vi "DLS_ERD Read.vi"(0 "GEA2 Reference In":refnum<k24>, 1 "Input Bit":T1, 2 "Co-efficient Data":T2, 5 "Standalone?":bool, 7 "GEA Inputs":T4 {"Destination" format="%.0x"; "Source" format="%.0x"}, 11 "Error In":errorcluster) -> (4 "GEA2 Reference Out":refnum<k24>, 6 "DLS ERD Data":T3, 8 "Result Q5 Tranformation":dbl, 15 "Error Out":errorcluster)   [LabVIEW 2016, in "TLMB.lvlib"]
doc: "This vi can be used to read ERD every 1 sec for user selected repeat counts."
uses:
  Projects/TLMB.lvlib
  Q:/Common/DLLs/GEA3/GeaCommunication.dll
  Common/DLLs/GEA3/GeaCommunication.dll
  Common/LabVIEW GEA2 Toolkit/LabVIEW_GEA2_Toolkit.lvlibp/type defs/Source_Destination.ctl
  Control/DLS ERD Data.ctl
  Common/LabVIEW GEA2 Toolkit/LabVIEW_GEA2_Toolkit.lvlibp/type defs/ERD Read Data In.ctl
  Common/LabVIEW GEA2 Toolkit/LabVIEW_GEA2_Toolkit.lvlibp/type defs/Data Type.ctl
  Common/LabVIEW GEA2 Toolkit/LabVIEW_GEA2_Toolkit.lvlibp
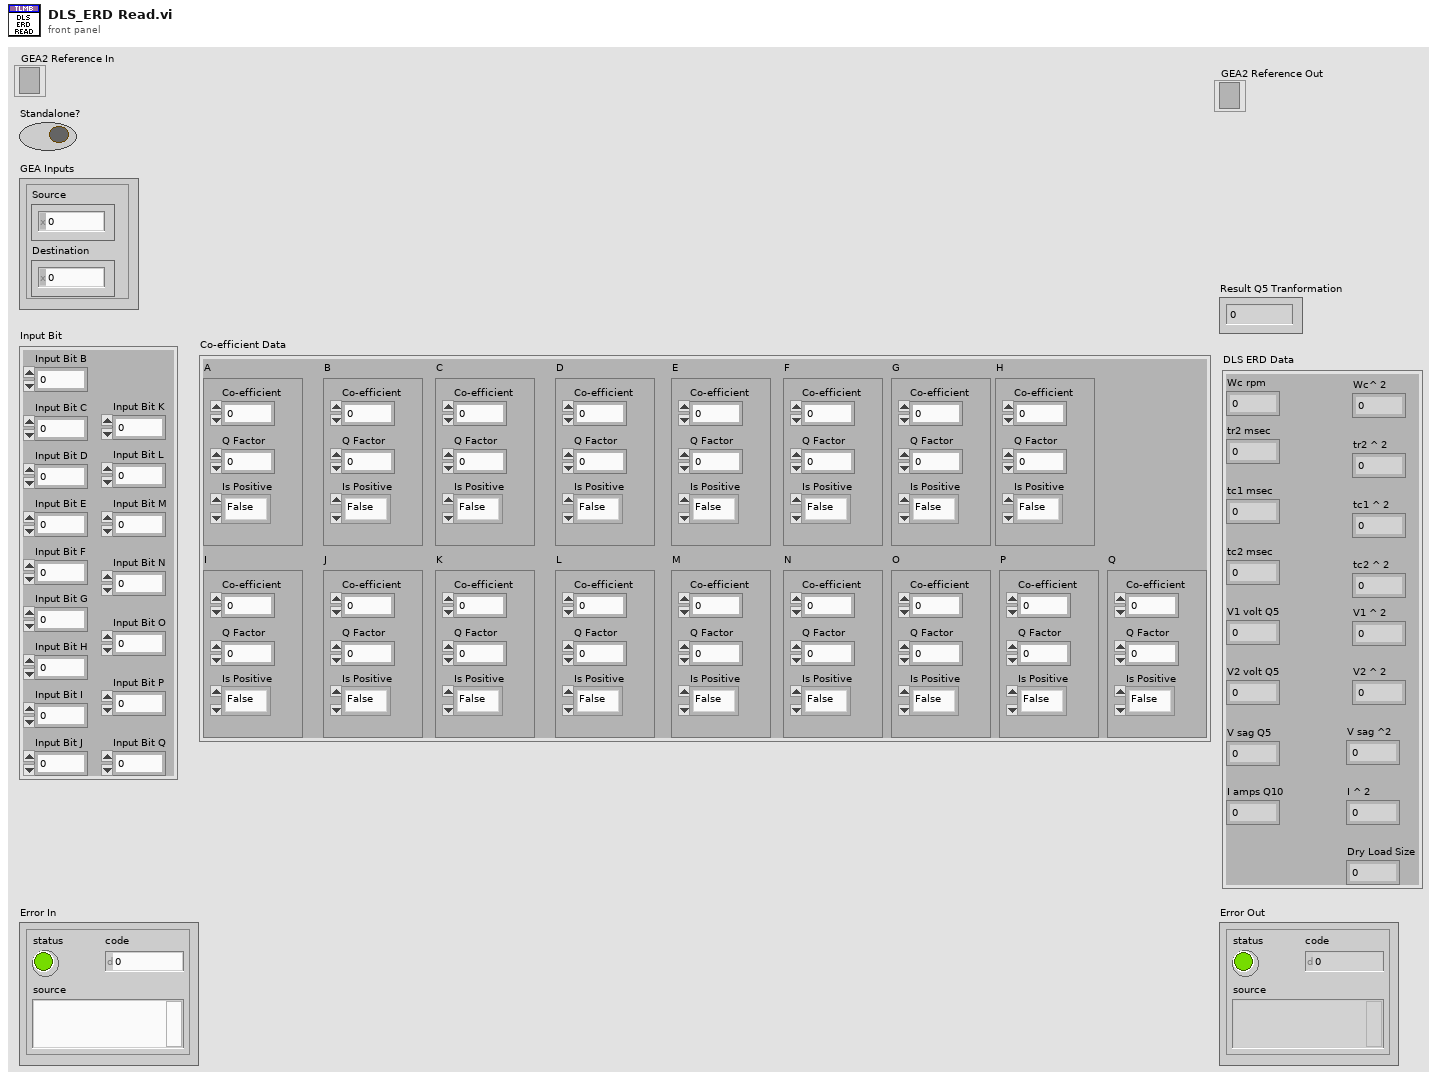
[diagram p1: front panel]
types:
  T1 = cluster{"Input Bit B":dbl, "Input Bit C":dbl, "Input Bit D":dbl, "Input Bit E":dbl, "Input Bit F":dbl, "Input Bit G":dbl, "Input Bit H":dbl, "Input Bit I":dbl, "Input Bit J":dbl, "Input Bit K":dbl, "Input Bit L":dbl, "Input Bit M":dbl, "Input Bit N":dbl, "Input Bit O":dbl, "Input Bit P":dbl, "Input Bit Q":dbl}
  T2 = cluster{"A":cluster{"Co-efficient":dbl, "Q Factor":dbl, "Is Positive":enum16{"False", "True"}}, "B":cluster{"Co-efficient":dbl, "Q Factor":dbl, "Is Positive":enum16{"False", "True"}}, "C":cluster{"Co-efficient":dbl, "Q Factor":dbl, "Is Positive":enum16{"False", "True"}}, "D":cluster{"Co-efficient":dbl, "Q Factor":dbl, "Is Positive":enum16{"False", "True"}}, "E":cluster{"Co-efficient":dbl, "Q Factor":dbl, "Is Positive":enum16{"False", "True"}}, "F":cluster{"Co-efficient":dbl, "Q Factor":dbl, "Is Positive":enum16{"False", "True"}}, "G":cluster{"Co-efficient":dbl, "Q Factor":dbl, "Is Positive":enum16{"False", "True"}}, "H":cluster{"Co-efficient":dbl, "Q Factor":dbl, "Is Positive":enum16{"False", "True"}}, "I":cluster{"Co-efficient":dbl, "Q Factor":dbl, "Is Positive":enum16{"False", "True"}}, "J":cluster{"Co-efficient":dbl, "Q Factor":dbl, "Is Positive":enum16{"False", "True"}}, "K":cluster{"Co-efficient":dbl, "Q Factor":dbl, "Is Positive":enum16{"False", "True"}}, "L":cluster{"Co-efficient":dbl, "Q Factor":dbl, "Is Positive":enum16{"False", "True"}}, "M":cluster{"Co-efficient":dbl, "Q Factor":dbl, "Is Positive":enum16{"False", "True"}}, "N":cluster{"Co-efficient":dbl, "Q Factor":dbl, "Is Positive":enum16{"False", "True"}}, "O":cluster{"Co-efficient":dbl, "Q Factor":dbl, "Is Positive":enum16{"False", "True"}}, "P":cluster{"Co-efficient":dbl, "Q Factor":dbl, "Is Positive":enum16{"False", "True"}}, "Q":cluster{"Co-efficient":dbl, "Q Factor":dbl, "Is Positive":enum16{"False", "True"}}}
  T3 = typedef "TLMB.lvlib/DLS ERD Data.ctl" = cluster{"Wc rpm":dbl, "tr2 msec":dbl, "tc1 msec":dbl, "tc2 msec":dbl, "V1 volt Q5":dbl, "V2 volt Q5":dbl, "I amps Q10":dbl, "Wc^ 2":dbl, "tr2 ^ 2":dbl, "tc1 ^ 2":dbl, "tc2 ^ 2":dbl, "V1 ^ 2":dbl, "V2 ^ 2":dbl, "I ^ 2":dbl, "V sag Q5":dbl, "V sag ^2":dbl, "Dry Load Size":dbl}
  T4 = typedef "LabVIEW_GEA2_Toolkit.lvlibp/Source_Destination.ctl" = cluster{"Source":u8, "Destination":u8}
  T5 = typedef "LabVIEW_GEA2_Toolkit.lvlibp/ERD Read Data In.ctl" = cluster{"ERD Number":u16, "Data Type":T6}
  T6 = typedef "LabVIEW_GEA2_Toolkit.lvlibp/Data Type.ctl" = enum16{"string", "boolean", "uint8_t", "uint16_t", "uint32_t", "uint64_t", "int8_t", "int16_t", "int32_t", "int64_t"}
  T7 = typedef "LabVIEW_GEA2_Toolkit.lvlibp/ERD Read Data Out.ctl" = cluster{"ERD Number":u16, "Data":string}
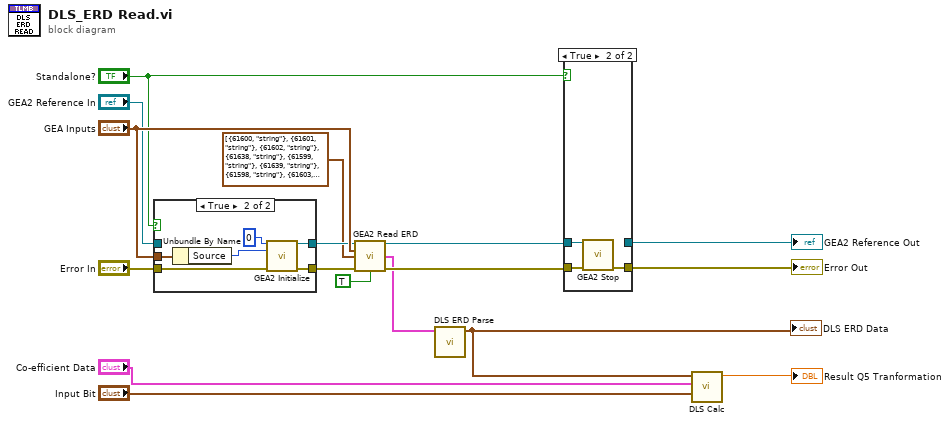
[diagram p0: block diagram]
diagram:
  n1 = case shown="True" "Standalone?" {
    tunnel: "Error In" -> [w18 w25]
    tunnel: [w18 w24] -> w12
    tunnel: "GEA2 Reference In" -> [w19 _]
    tunnel: [w19 w23] -> w11
    tunnel: "GEA Inputs" -> [_ w21]
    frame False {
    }
    frame True {
      n2 = Unbundle By Name(w21) -> ("Source"=w22:u8)
      n3 = call "GEA2 Initialize.vi"("Board Index"=0, "Source Address"=w22, "error in"=w25) -> ("GEA2 Reference Out"=w23:refnum<k24>, "error out"=w24:errorcluster)  [unwired: 10 in, 1 out]
    }
  }
  n4 = call "GEA2 Read ERD.vi"("GEA2 Reference In"=w11, "GEA Inputs"="GEA Inputs", "Read ERD List"=T5[] [{"ERD Number"=61600, "Data Type"=enum."string"}, {"ERD Number"=61601, "Data Type"=enum."string"}, {"ERD Number"=61602, "Data Type"=enum."string"}, {"ERD Number"=61638, "Data Type"=enum."string"}, {"ERD Number"=61599, "Data Type"=enum."string"}, {"ERD Number"=61639, "Data Type"=enum."string"}, {"ERD Number"=61598, "Data Type"=enum."string"}, {"ERD Number"=61603, "Data Type"=enum."string"}], "Error In"=w12, "Verify ERD Response?"=TRUE) -> ("GEA2 Reference Out"=w8:refnum<k24>, "ERD Data Out"=w6:T7[], "Error Out"=w9:errorcluster)  [unwired: 7 in, 1 out]
  n5 = call "DLS ERD Parse.vi"("ERD Data Out"=w6) -> ("DLS ERD Data 2"=w2:T3)  [unwired: 10 in]
  "DLS ERD Data" <- w2
  n6 = case shown="True" "Standalone?" {
    tunnel: w9 -> [w26 w29]
    tunnel: [w26 w28] -> w16
    tunnel: w8 -> [w27 w30]
    tunnel: [w27 _] -> w10
    frame False {
    }
    frame True {
      n7 = call "GEA2 Stop.vi"("GEA2 Reference In"=w30, "Error In"=w29) -> ("Error Out"=w28:errorcluster)  [unwired: 13 in]
    }
  }
  "Error Out" <- w16
  "GEA2 Reference Out" <- w10
  n8 = call "DLS Calc.vi"("Input Bit"="Input Bit", "Coeff Data"="Co-efficient Data", "DLS ERD Data"=w2) -> ("Result Q5 Tranformation"=→"Result Q5 Tranformation":dbl)  [unwired: 8 in]
